vi "check_base_folder.vi"(8 "error in":errorcluster, 11 "reference cluster in":T1) -> (0 "error out":errorcluster, 3 "reference cluster out":T1, 4 "directory out":path=path "C:/Users/training/Desktop/Data")   [LabVIEW 2016]
uses:
  Type Definitions/reference_cluster.ctl
  Type Definitions/vars_settings.ctl
  Type Definitions/stim_type.ctl
  Type Definitions/vars_runtime.ctl
  Type Definitions/data.ctl
  Type Definitions/notifier_elements_GUI.ctl
  Type Definitions/notifier_elements_DAQ.ctl
  Type Definitions/notifier_elements_write.ctl
  Type Definitions/control_references.ctl
  <vilib>/Utility/sysdir.llb/System Directory Type.ctl
  <userlib>/_OpenG.lib/file/file.llb/Strip Path - Traditional__ogtk.vi
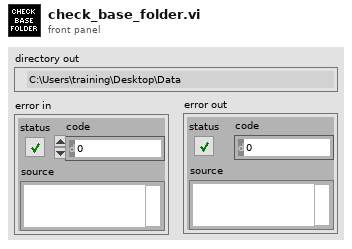
[diagram p1: front panel]
types:
  T1 = typedef "reference_cluster.ctl" = cluster{"Vars":cluster{"General":refnum<notifier>, "Runtime":refnum<notifier>}, "Data":cluster{"Display":refnum<queue>, "Write":refnum<queue>}, "LoopCtrl":cluster{"Display":refnum<notifier>, "DAQ":refnum<notifier>, "Write":refnum<notifier>[]}, "Controls":T2, "Error Notifier":refnum<notifier>}
  T2 = typedef "control_references.ctl" = cluster{"Base Directory":refnum<vi>, "Config File":refnum<vi>, "Timing Issues":refnum<vi>, "Quit":refnum<vi>, "Animal ID":refnum<vi>[], "Session ID":refnum<vi>[], "Active":refnum<vi>[], "Temperature Charts":refnum<vi>[], "Lick Charts":refnum<vi>[], "Bool Displays":refnum<vi>[], "Stimulus Timing":refnum<vi>[], "Stimulus Stats":refnum<vi>[], "Catch Stats":refnum<vi>[], "Recording Status":refnum<vi>[]}
  T3 = typedef "System Directory Type.ctl" = i32
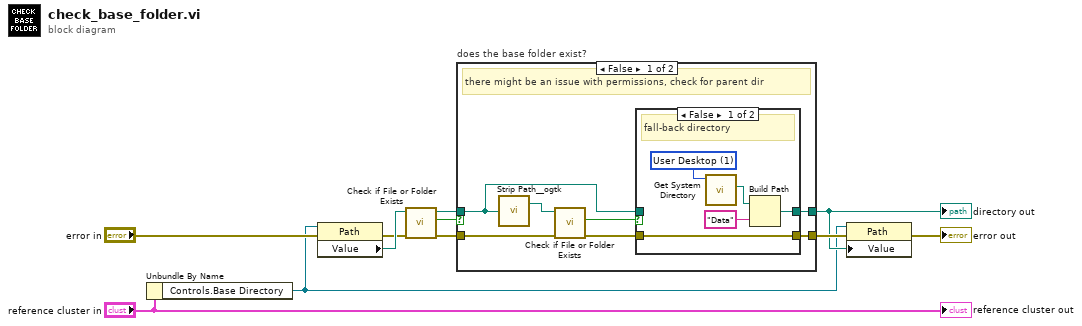
[diagram p0: block diagram]
diagram:
  n1 = Unbundle By Name("reference cluster in") -> ("Controls.Base Directory"=w2:refnum<vi>)
  n2 = property class="Path"(reference=w2, error in="error in") -> (error out=w6:errorcluster, "Value"=w8:path)  [unwired: 1 out]
  n3 = call <vilib>:"Check if File or Folder Exists.vi"("error in (no error)"=w6, "path"=w8) -> ("error out"=w9:errorcluster, "file or folder exists?"=w11:bool, "dup path"=w10:path)  [unwired: 7 in]
  n4 = case "does the base folder exist?" shown="False" w11 {
    tunnel: w10 -> [w14 w26]
    tunnel: w9 -> [w18 w27]
    tunnel: [w12 w27] -> w5
    tunnel: [w13 w26] -> w3
    frame False {
      # "there might be an issue with permissions, check for parent dir"
      n5 = call-poly <userlib>:"Strip Path__ogtk.vi"("path"=w14) -> ("stripped path"=w17:path)  [unwired: 1 out]
      n6 = call <vilib>:"Check if File or Folder Exists.vi"("error in (no error)"=w18, "path"=w17) -> ("error out"=w16:errorcluster, "file or folder exists?"=w15:bool)  [unwired: 7 in, 1 out]
      n7 = case shown="False" w15 {
        tunnel: w16 -> [w22 w24]
        tunnel: w14 -> [_ w25]
        tunnel: [w20 w25] -> w13
        tunnel: [w22 w24] -> w12
        frame False {
          w23 = T3 1 items=["User Home"=0, "User Desktop"=1, "User Documents"=2, "User Application Data"=3, "User Preferences"=4, "User Temporary"=5, "Public Documents"=6, "Public Application Data"=7, "Public Preferences"=8, "Public Cache"=13, "System Core Libraries"=9, "System Installed Libraries"=10, "Application Files"=11, "Boot Volume Root"=12] ("system directory type")
          # "fall-back directory"
          n8 = call <vilib>:"Get System Directory.vi"("system directory type"=w23) -> ("system directory"=w21:path)  [unwired: 10 in]
          n9 = Build Path(base path=w21, name or relative path="Data") -> (appended path=w20:path)
        }
        frame True {
          # "all good ... carry on"
        }
      }
    }
    frame True {
      # "all good ... carry on"
    }
  }
  "directory out" <- w3
  n10 = property class="Path"(reference=w2, error in=w5, "Value"=w3) -> (error out=→"error out":errorcluster)  [unwired: 1 out]
  "reference cluster out" <- "reference cluster in"
